vi "ControlToCommand.vi"   [LabVIEW 2020, in "TextControlledInstrum.lvlib"]
uses:
  TextControlledInstrum.lvlib
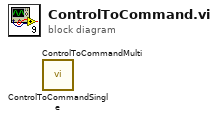
[diagram p0: block diagram]
diagram:
  n1 = call "ControlToCommandSingle.vi"() -> ()  [unwired: 11 in, 1 out]
  n2 = call "ControlToCommandMulti.vi"() -> ()  [unwired: 11 in, 1 out]
